vi "sub_ImageProcess.vi"(0 "참조 번호 입력":T1, 1 "Range":cluster{"Lower value":sgl, "Upper value":sgl}={"Lower value"=128.0, "Upper value"=255.0} {"Upper value" format="%.2f"; "Lower value" format="%.2f"}, 3 "ROI":T3, 5 "배열":T1[](array[typedef]), 7 "클러스터":T5, 9 "Local":T4, 11 "에러 입력(에러 없음)":errorcluster) -> (4 "참조 번호 출력":T1, 6 "Number of Particles":i32, 10 "Particle Reports (Pixels)":T2(array[cluster]), 15 "error out":errorcluster)   [LabVIEW 2014]
uses:
  <vilib>/vision/Image Controls.llb/IMAQ Image.ctl
  <vilib>/vision/NI_Vision_Development_Module.lvlib
panel:
  out "웨이브폼 그래프":dbl[](graph)
  out "최소값":dbl
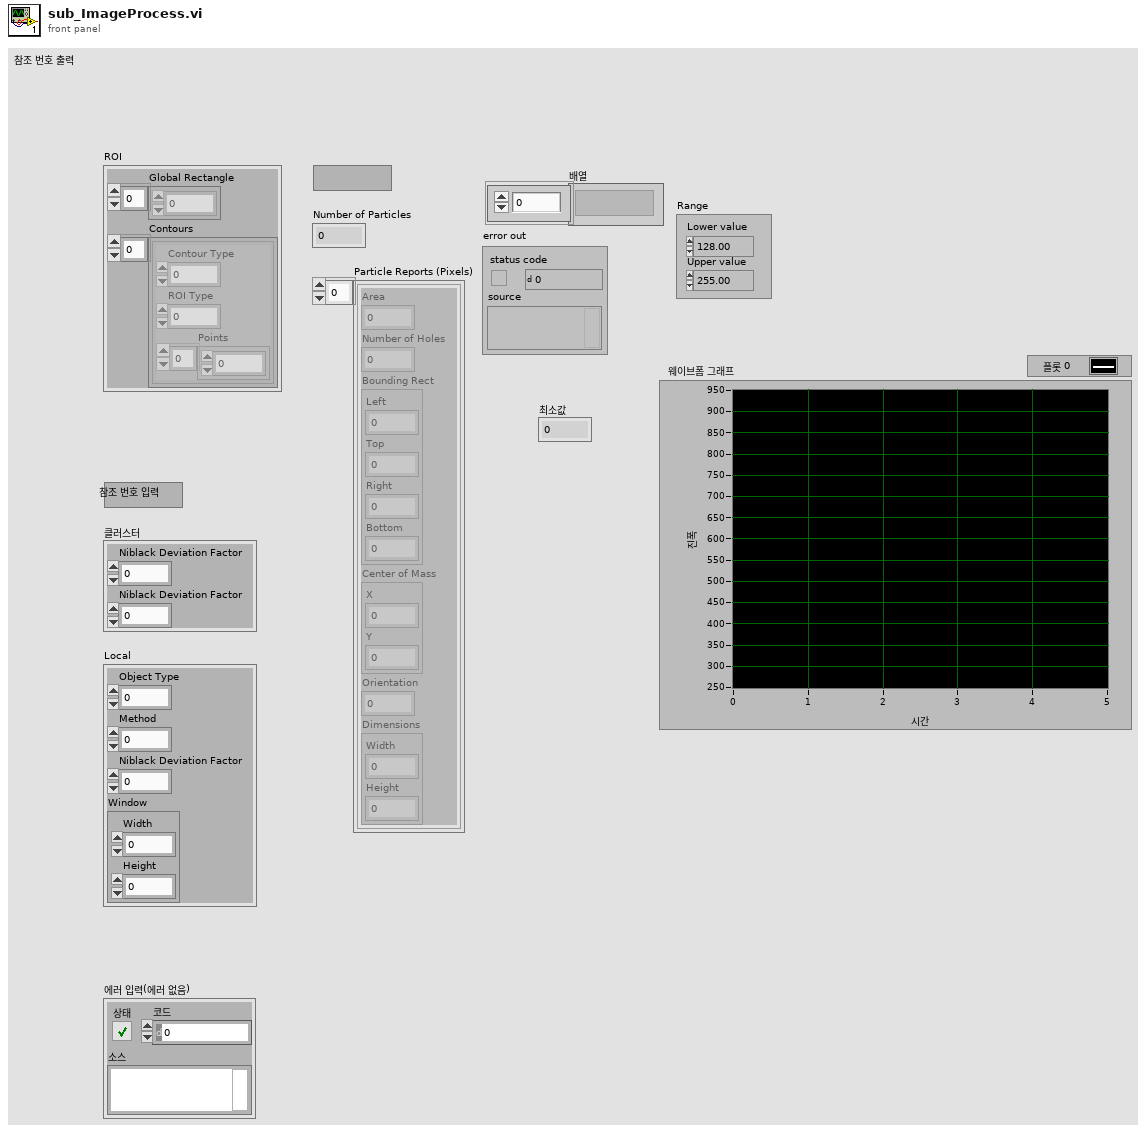
[diagram p1: front panel]
types:
  T1 = typedef "IMAQ Image.ctl" = refnum<image>
  T2 = cluster{"Area":dbl, "Number of Holes":dbl, "Bounding Rect":cluster{"Left":dbl, "Top":dbl, "Right":dbl, "Bottom":dbl}, "Center of Mass":cluster{"X":dbl, "Y":dbl}, "Orientation":dbl, "Dimensions":cluster{"Width":dbl, "Height":dbl}}[]
  T3 = cluster{"Global Rectangle":i32[], "Contours":cluster{"Contour Type":u32, "ROI Type":u32, "Points":i32[]}[]}
  T4 = cluster{"Object Type":u32, "Method":u32, "Niblack Deviation Factor":dbl, "Window":cluster{"Width":i32, "Height":i32}}
  T5 = cluster{"Niblack Deviation Factor":dbl, "Niblack Deviation Factor":dbl}
  T6 = enum32{"AutoM", "Close", "Dilate", "Erode", "Gradient", "Gradient out", "Gradient in", "Hit miss", "Open", "PClose", "POpen", "Thick", "Thin"}
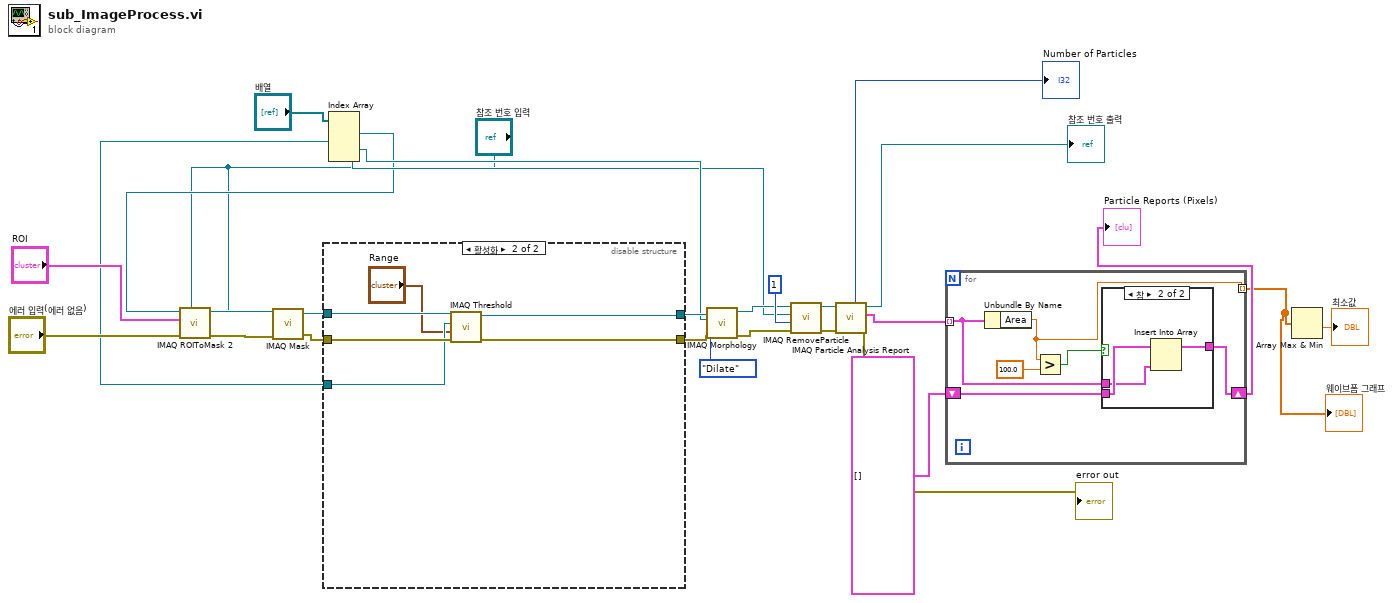
[diagram p0: block diagram]
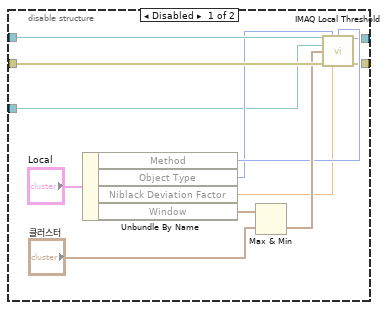
[diagram p2: hidden frame]
diagram:
  n1 = Index Array(array="배열") -> (element #1=w2:T1, element #2=w16:T1, element #3=w9:T1, element #4=w8:T1)  [unwired: 4 in]
  n2 = call "IMAQ ROIToMask 2"("Image Model"="참조 번호 입력", "error in (no error)"="에러 입력(에러 없음)", "ROI Descriptor"="ROI", "Image"=w2) -> ("error out"=w24:errorcluster, "Image Out"=w25:T1)  [unwired: 5 in, 1 out]
  n3 = call "IMAQ Mask"("error in (no error)"=w24, "Image Mask"=w25, "Image Src"="참조 번호 입력") -> ("error out"=w27:errorcluster, "Image Dst Out"=w20:T1)  [unwired: 2 in]
  n4 = disable-structure shown="활성화" {
    disable-tunnel: w27 -> [w40 w44]
    disable-tunnel: w20 -> [w39 w46]
    disable-tunnel: w16 -> [w31 w42]
    disable-tunnel: [w30 w45] -> w14
    disable-tunnel: [w29 w43] -> w12
    frame Disabled {
      n5 = Unbundle By Name("Local") -> ("Method"=w34:u32, "Object Type"=w33:u32, "Niblack Deviation Factor"=w32:dbl, "Window"=w36:cluster{"Width":i32, "Height":i32})
      n6 = Max & Min(x=w36, y="클러스터") -> (min(x,y)=w35:cluster{dbl, dbl})  [unwired: 1 out]
      n7 = call "IMAQ Local Threshold"("Image Src"=w39, "Look For (Bright Objects)"=w33, "Method (Niblack)"=w34, "Image Dst"=w31, "Window Size (32x32)"=w35, "error in (no error)"=w40, "Niblack Deviation Factor (0.2)"=w32) -> ("Image Dst Out"=w30:T1, "error out"=w29:errorcluster)  [unwired: 7 in]
    }
    frame Enabled {
      n8 = call "IMAQ Threshold"("error in (no error)"=w44, "Range"="Range", "Image Dst"=w42, "Image Src"=w46) -> ("error out"=w43:errorcluster, "Image Dst Out"=w45:T1)  [unwired: 6 in]
    }
  }
  n9 = call "IMAQ Morphology"("error in (no error)"=w12, "Operation"=T6."Dilate", "Image Dst"=w9, "Image Src"=w14) -> ("error out"=w11:errorcluster, "Image Dst Out"=w13:T1)  [unwired: 6 in]
  n10 = call "IMAQ RemoveParticle"("error in (no error)"=w11, "Number of Erosion"=1, "Image Dst"=w8, "Image Src"=w13) -> ("error out"=w22:errorcluster, "Image Dst Out"=w21:T1)  [unwired: 6 in]
  n11 = call "IMAQ Particle Analysis Report"("error in (no error)"=w22, "Image"=w21) -> ("error out"=→"error out":errorcluster, "Particle Reports (Pixels)"=w7:T2, "Image Out (duplicate)"=→"참조 번호 출력":T1, "Number of Particles"=→"Number of Particles":i32)  [unwired: 4 in, 2 out]
  n12 = for {
    tunnel: w7 -> [w49] mode=indexing
    shift-right: [w50] -> w5
    shift-left: T2 [] -> [w51]
    tunnel: [w47] -> w3 mode=indexing
    n13 = Unbundle By Name(w49) -> ("Area"=w47:dbl)
    n14 = Greater?(x=w47, y=100.0) -> (0:w52:bool)
    n15 = case shown="참" w52 {
      tunnel: w51 -> [w53 w56]
      tunnel: [w53 w55] -> w50
      tunnel: w49 -> [_ w54]
      frame False {
      }
      frame True {
        n16 = Insert Into Array(array=w56, new element=w54) -> (w55:T2)  [unwired: 1 in]
      }
    }
  }
  "Particle Reports (Pixels)" <- w5
  "웨이브폼 그래프" <- w3
  n17 = Array Max & Min(array=w3) -> (min value=→"최소값":dbl)  [unwired: 3 out]
